vi "状态号.vi"() -> ()   [LabVIEW 2013]
uses:
  S7Ref.vi
panel:
  out "error out 2":errorcluster
  in  "写入地址":u32=1000
  in  "error in (no error)":errorcluster
  out "error out":errorcluster
  out "状态":bool
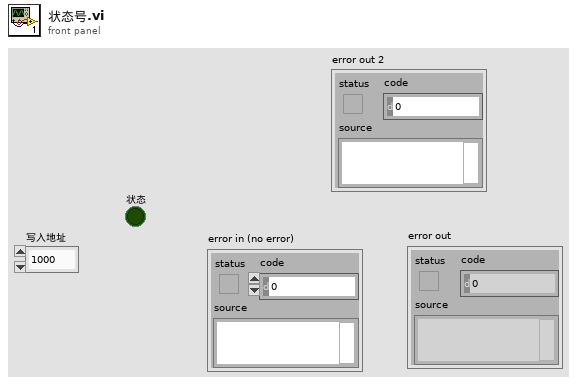
[diagram p1: front panel]
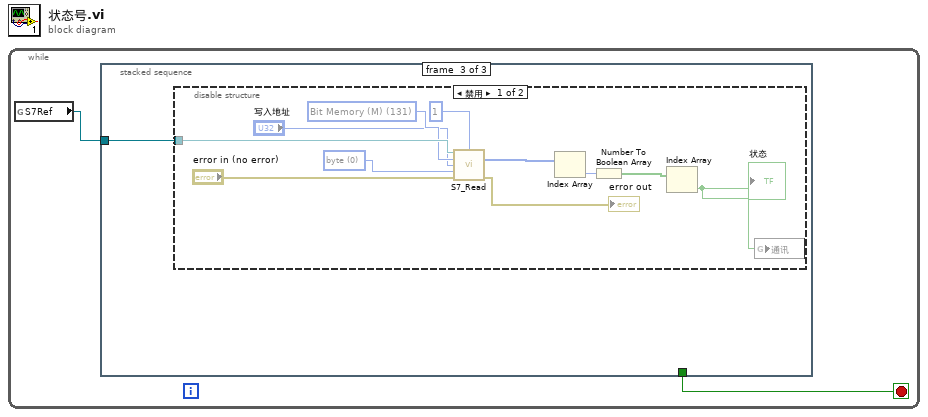
[diagram p0: block diagram]
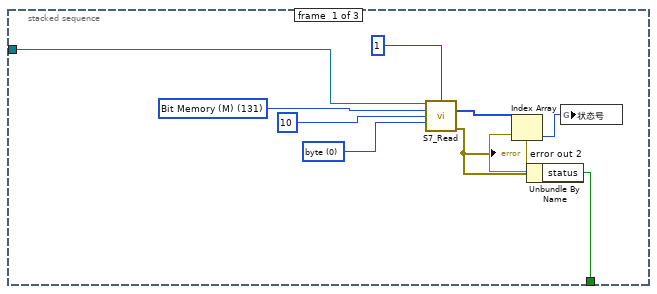
[diagram p2: hidden frame]
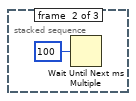
[diagram p3: hidden frame]
diagram:
  n1 = while {
    stop <- w1 stop-if-true
    n2 = global read "S7Ref.vi" "S7Ref"() -> (w2:refnum<k5>)
    n3 = stacked-sequence {
      tunnel: w2 -> [w11 _ w13]
      tunnel: [w10 _ _] -> w1
      frame #0 {
        w6 = u16 0 items=["byte", "word", "Dword"] ("数据类型")
        w8 = u8 131 items=["I/O (P)"=128, "Input (I)"=129, "Output (Q)"=130, "Bit Memory (M)"=131, "Data (DB)"=132, "Instance Data (DI)"=133, "Local Data (L)"=134, "Predecessor Local Data (VL)"=135] ("寄存器类型")
        n4 = call "S7_Read .vi"("TCP"=w11, "读取长度"=u16 1, "寄存器类型"=w8, "起始地址"=u32 10, "数据类型"=w6) -> ("数据"=w9:u32[], "error out"=w4:errorcluster)  [unwired: 7 in, 2 out]
        "error out 2" <- w4
        n5 = Index Array(array=w9) -> (element=w3:u32)  [unwired: 1 in]
        n6 = Unbundle By Name(w4) -> ("status"=w10:bool)
        n7 = global write "全局 1.vi" "状态号"(w3) -> ()
      }
      frame #1 {
        n8 = Wait Until Next ms Multiple(millisecond multiple=u32 100 ("毫秒倍数")) -> ()  [unwired: 1 out]
      }
      frame #2 {
        n9 = disable-structure shown="禁用" {
          disable-tunnel: w13 -> [w24 _]
          frame Disabled {
            w19 = u16 0 items=["byte", "word", "Dword"] ("数据类型")
            w21 = u8 131 items=["I/O (P)"=128, "Input (I)"=129, "Output (Q)"=130, "Bit Memory (M)"=131, "Data (DB)"=132, "Instance Data (DI)"=133, "Local Data (L)"=134, "Predecessor Local Data (VL)"=135] ("寄存器类型")
            n10 = call "S7_Read .vi"("TCP"=w24, "读取长度"=u16 1, "寄存器类型"=w21, "起始地址"="写入地址", "数据类型"=w19, "error in"="error in (no error)") -> ("数据"=w22:u32[], "error out"=→"error out":errorcluster)  [unwired: 6 in, 2 out]
            n11 = Index Array(array=w22) -> (element=w18:u32)  [unwired: 1 in]
            n12 = Number To Boolean Array(number=w18) -> (Boolean array=w23:bool[])
            n13 = Index Array(array=w23) -> (element=w15:bool)  [unwired: 1 in]
            "状态" <- w15
            n14 = global write "全局 1.vi" "通讯"(w15) -> ()
          }
          frame Enabled {
          }
        }
      }
    }
  }
